vi "Simple Solenoid Controller.vi"(8 "error in (no error)":errorcluster, 9 "Reverse":bool, 10 "Forward":bool, 11 "refnum name":string) -> (0 "error out":errorcluster, 3 "Set To":T1)   [LabVIEW 2011]
uses:
  <vilib>/Rock Robotics/WPI/Solenoid/WPI_SolenoidValue.ctl
  <vilib>/Rock Robotics/WPI/Solenoid/WPI_SolenoidSetEnum.vi
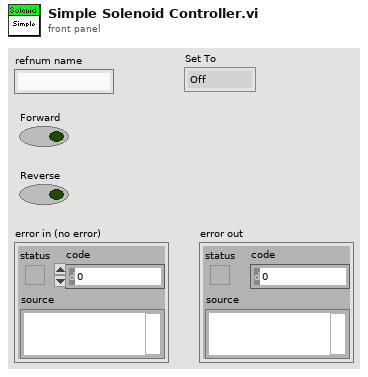
[diagram p1: front panel]
types:
  T1 = typedef "WPI_SolenoidValue.ctl" = enum16{"Off", "On", "Forward", "Reverse"}
  T2 = typedef "WPI_SolenoidDevRef.ctl" = cluster{"DevStatus":errorcluster, "Solenoid Module":T3, "Forward Solenoid Channel":T4, "Reverse Solenoid Channel":T4}
  T3 = typedef "FPGA_TypedefSolenoidModule.ctl" = enum16{"Solenoid Module 1", "Solenoid Module 2"}
  T4 = typedef "WPI_SolenoidChannel.ctl" = enum8{"Solenoid 1", "Solenoid 2", "Solenoid 3", "Solenoid 4", "Solenoid 5", "Solenoid 6", "Solenoid 7", "Solenoid 8", "Invalid"}
  T5 = typedef "WPI_RelayDevRef.ctl" = cluster{"DevStatus":errorcluster, "Relay Channel":T6, "Digital Module":T7, "Relay Direction":T8}
  T6 = typedef "FPGA_DIORelayChannel.ctl" = enum8{"Relay 1", "Relay 2", "Relay 3", "Relay 4", "Relay 5", "Relay 6", "Relay 7", "Relay 8", "Invalid"}
  T7 = typedef "FPGA_TypedefDigitalModule.ctl" = enum16{"Digital Module 1", "Digital Module 2"}
  T8 = typedef "WPI_RelayDirection.ctl" = enum16{"Both directions", "Forward only", "Reverse only"}
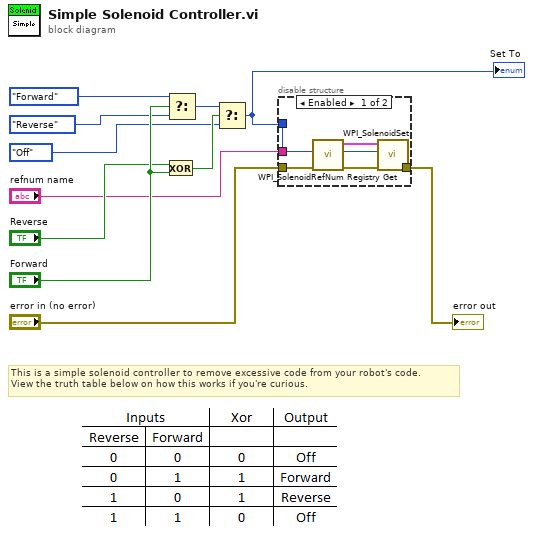
[diagram p0: block diagram]
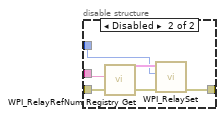
[diagram p2: hidden frame]
diagram:
  # "This is a simple solenoid controller to remove excessive code from your robot's code.\nView the truth table below on how this works if you're curious."
  n1 = Exclusive Or(1:"Forward", 2:"Reverse") -> (0:w9:bool)
  n2 = Select(t=WPI_SolenoidValue."Forward" ("Value"), s="Forward", f=WPI_SolenoidValue."Reverse" ("Value")) -> (s? t:f=w2:T1)
  n3 = Select(t=w2, s=w9, f=WPI_SolenoidValue."Off" ("t")) -> (s? t:f=w6:T1)
  "Set To" <- w6
  n4 = disable-structure shown="Enabled" {
    disable-tunnel: [w17 w22] -> w11
    disable-tunnel: "error in (no error)" -> [w16 w23]
    disable-tunnel: w6 -> [w15 w18]
    disable-tunnel: "refnum name" -> [w12 w19]
    frame Enabled {
      n5 = call <vilib>:"WPI_SolenoidRefNum Registry Get.vi"("error in (no error)"=w16, "refnum name"=w12) -> ("error out"=w14:errorcluster, "SolenoidDevRef"=w13:T2)  [unwired: 8 in]
      n6 = call-poly <vilib>:"WPI_SolenoidSet.vi"("error in (no error)"=w14, "Value"=w15, "SolenoidDevRef"=w13) -> ("error out"=w17:errorcluster)  [unwired: 7 in, 1 out]
    }
    frame Disabled {
      n7 = call <vilib>:"WPI_RelayRefNum Registry Get.vi"("error in (no error)"=w23, "refnum name"=w19) -> ("error out"=w21:errorcluster, "RelayDevRef"=w20:T5)  [unwired: 8 in]
      n8 = call <vilib>:"WPI_RelaySet.vi"("error in (no error)"=w21, "RelayValue"=w18, "RelayDevRef"=w20) -> ("error out"=w22:errorcluster)  [unwired: 7 in, 1 out]
    }
  }
  "error out" <- w11
